vi "Initialize.vi"(8 "error in (no error)":errorcluster, 10 "Opciones puerto":T1={"baud rate (9600)"=9600, "data bits (8)"=8, "parity (0:none)"=enum."None"} {"data bits (8)" min=5 max=8 step=1}, 11 "Puerto Serial":refnum<visa-resource-name>) -> (0 "error out":errorcluster, 2 "Connected?":bool, 3 "VISA resource name out":refnum<visa-resource-name>)   [LabVIEW 2020, in "Control de MaP.lvlib"]
doc: "Establece la comunicación con el instrumento"
uses:
  Control de MaP.lvlib
  Controls/Com Port Options.ctl
  <vilib>/Instr/_visa.llb/VISA Flush IO Buffer Mask.ctl
  <vilib>/Instr/_visa.llb/VISA Configure Serial Port (Instr).vi
panel:
  # "Centro de investigaciones en óptica.  ALL RIGHTS RESERVED."
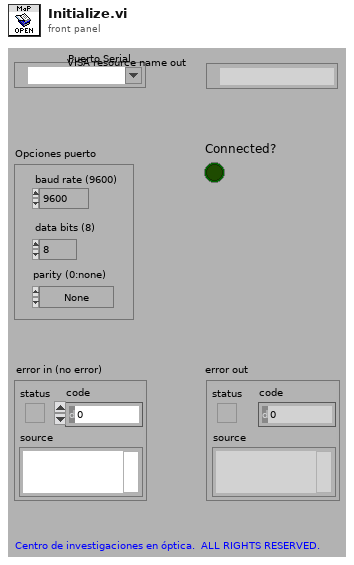
[diagram p1: front panel]
types:
  T1 = typedef "Control de MaP.lvlib/Com Port Options.ctl" = cluster{"baud rate (9600)":u32, "data bits (8)":u16, "parity (0:none)":enum16{"None", "Odd", "Even", "Mark", "Space"}}
  T2 = typedef "VISA Flush IO Buffer Mask.ctl" = u16
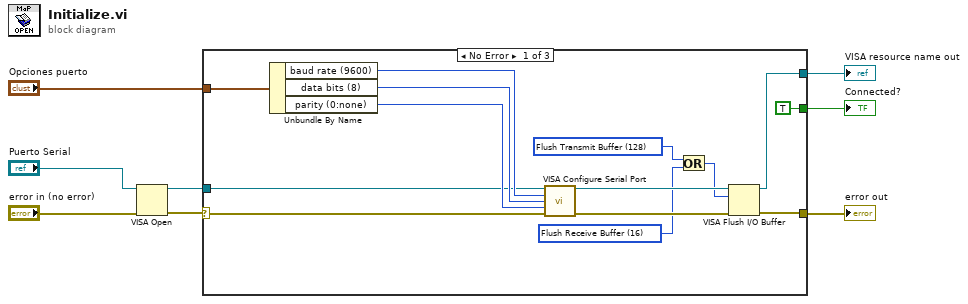
[diagram p0: block diagram]
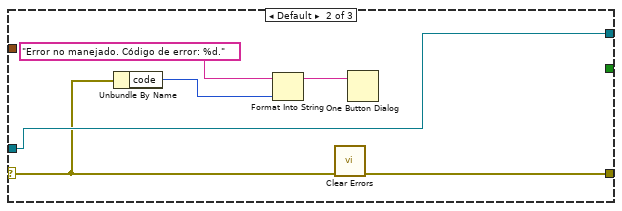
[diagram p2: hidden frame]
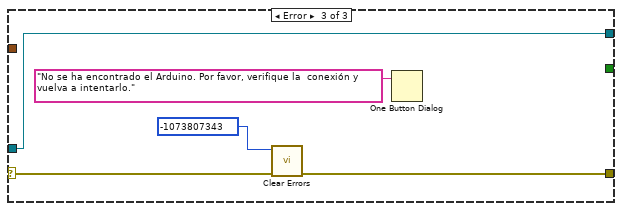
[diagram p3: hidden frame]
diagram:
  n1 = VISA Open(error in (no error)="error in (no error)", VISA resource name="Puerto Serial") -> (VISA resource name=w5:refnum<visa-resource-name>, error out=w3:errorcluster)  [unwired: 3 in]
  n2 = case shown="No Error" w3 {
    selector: w3 -> [w9 w26 w31]
    tunnel: [w17 w28 w33] -> w8
    tunnel: [w18 w27 w29] -> w7
    tunnel: "Opciones puerto" -> [w22 _ _]
    tunnel: w5 -> [w11 w28 w33]
    tunnel: [TRUE _ _] -> w1
    frame No Error {
      w12 = T2 16 items=["Flush Receive Buffer"=16, "Write Transmit Buffer to Device"=32, "Flush Receive Buffer (No I/O)"=64, "Flush Transmit Buffer"=128] ("Mask")
      w14 = T2 128 items=["Flush Receive Buffer"=16, "Write Transmit Buffer to Device"=32, "Flush Receive Buffer (No I/O)"=64, "Flush Transmit Buffer"=128] ("Mask")
      n3 = Unbundle By Name(w22) -> ("baud rate (9600)"=w21:u32, "data bits (8)"=w20:u16, "parity (0:none)"=w19:enum16{"None", "Odd", "Even", "Mark", "Space"})
      n4 = call-poly "VISA Configure Serial Port"("VISA resource name"=w11, "baud rate (9600)"=w21, "data bits (8)"=w20, "parity (0:none)"=w19, "error in (no error)"=w9) -> ("VISA resource name out"=w16:refnum<visa-resource-name>, "error out"=w15:errorcluster)  [unwired: 9 in]
      n5 = Or(x=w14, y=w12) -> (x .or. y?=w13:T2)
      n6 = VISA Flush I/O Buffer(VISA resource name=w16, mask (16)=w13, error in (no error)=w15) -> (VISA resource name out=w17:refnum<visa-resource-name>, error out=w18:errorcluster)
    }
    frame Default {
      n7 = Unbundle By Name(w26) -> ("code"=w24:i32)
      n8 = Format Into String(initial string="Error no manejado. Código de error: %d.", w24) -> (resulting string=w23:string)  [unwired: 2 in, 1 out]
      n9 = call <vilib>:"Clear Errors.vi"("error in (no error)"=w26) -> ("error out"=w27:errorcluster)  [unwired: 5 in, 1 out]
      n10 = One Button Dialog(message=w23) -> ()  [unwired: 1 in, 1 out]
    }
    frame Error {
      n11 = call <vilib>:"Clear Errors.vi"("error in (no error)"=w31, "specific error code to clear (0: all)"=-1073807343) -> ("error out"=w29:errorcluster)  [unwired: 4 in, 1 out]
      n12 = One Button Dialog(message="No se ha encontrado el Arduino. Por favor, verifique la  conexión y vuelva a intentarlo.") -> ()  [unwired: 1 in, 1 out]
    }
  }
  "VISA resource name out" <- w8
  "error out" <- w7
  "Connected?" <- w1
